vi "emergency stop.vi"() -> ()   [LabVIEW 2020]
panel:
  in  "emergency stop":bool
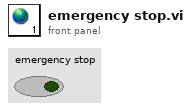
[diagram p1: front panel]
diagram:
